vi "Custom Device State to String.vi"(7 "Initialized?":bool) -> (8 "Custom Device State":string)   [LabVIEW 2020, in "SLSC EDS System Explorer.lvlib"]
uses:
  SLSC EDS System Explorer.lvlib
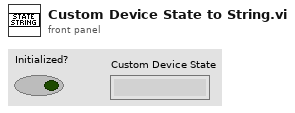
[diagram p1: front panel]
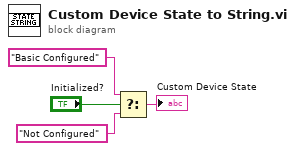
[diagram p0: block diagram]
diagram:
  n1 = Select(t="Basic Configured", s="Initialized?", f="Not Configured") -> (s? t:f=→"Custom Device State":string)
